vi "Convert DTCs.vi"(11 "value":T2 {"payload" format="%x"; "timestamp" format="%<%.7X\n%x>T"; "type" items=["CAN Data"=0, "CAN Remote"=1, "CAN Bus Error"=2, "CAN 2.0 Data"=8, "CAN FD Data"=16, "CAN FD+BRS Data"=24, "J1939 Data"=192, "Delay"=224, "Log Trigger"=225, "Start Trigger"=226]; "identifier" format="%x"}) -> (3 "Cluster":T1)   [LabVIEW 2015, in "J1939 Addon Shared.lvlib"]
uses:
  J1939 Addon Shared.lvlib
  <vilib>/xnet/xnet.llb/XNET Frame CAN.ctl
  <vilib>/xnet/xnet.llb/XNET Frame Type CAN.ctl
  Types/Convert DTCs Cluster.ctl
  J1939 Utilities/SubVIs/Convert CAN Arb ID to J1939 ID.vi
  J1939 Utilities/J1939 Utilities.lvlib
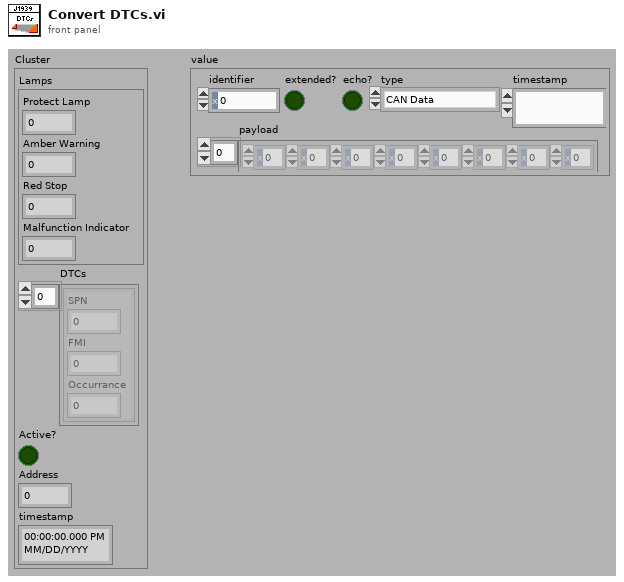
[diagram p1: front panel]
types:
  T1 = typedef "J1939 Addon Shared.lvlib/Convert DTCs Cluster.ctl" = cluster{"Lamps":cluster{"Protect Lamp":u8, "Amber Warning":u8, "Red Stop":u8, "Malfunction Indicator":u8}, "DTCs":cluster{"SPN":u32, "FMI":u8, "Occurrance":u8}[], "Active?":bool, "Address":u8, "timestamp":timestamp}
  T2 = typedef "XNET Frame CAN.ctl" = cluster{"timestamp":timestamp, "payload":u8[], "identifier":u32, "type":T3, "extended?":bool, "echo?":bool}
  T3 = typedef "XNET Frame Type CAN.ctl" = u8
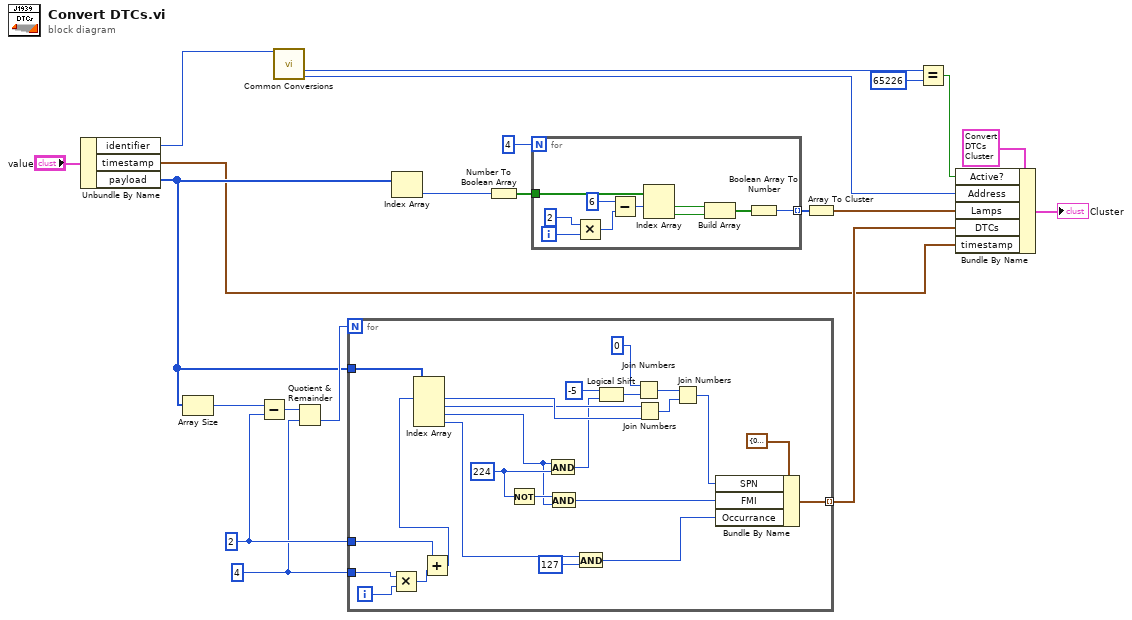
[diagram p0: block diagram]
diagram:
  w10 = 4 ("x")
  w12 = 2 ("x")
  n1 = Unbundle By Name("value") -> ("identifier"=w6:u32, "timestamp"=w1:timestamp, "payload"=w7:u8[])
  n2 = Array Size(array=w7) -> (size(s)=w13:i32)
  n3 = Subtract(x=w13, y=w12) -> (x-y=w11:i32)
  n4 = call-poly "Common Conversions.vi"("Arb ID"=w6) -> ("PGN"=w5:u32, "Source Address"=w2:u8)  [unwired: 11 in, 2 out]
  n5 = Quotient & Remainder(x=w11, y=w10) -> (floor(x/y)=w9:i32)  [unwired: 1 out]
  n6 = for {
    N: w9 -> [_]
    tunnel: w7 -> [w45]
    tunnel: [w30] -> w15 mode=indexing
    tunnel: w12 -> [w26]
    tunnel: w10 -> [w25]
    i -> [w29]
    w39 = u8 224 ("y")
    n7 = Multiply(x=w25, y=w29) -> (x*y=w28:i32)
    n8 = Add(x=w26, y=w28) -> (x+y=w27:i32)
    n9 = Index Array(array=w45, index #1=w27) -> (element #1=w41:u8, element #2=w40:u8, element #3=w37:u8, element #4=w36:u8)  [unwired: 3 in]
    n10 = Not(x=w39) -> (.not. x?=w38:u8)
    n11 = And(x=w37, y=w39) -> (x .and. y?=w23:u8)
    n12 = And(x=w38, y=w37) -> (x .and. y?=w32:u8)
    n13 = And(x=w36, y=u8 127) -> (x .and. y?=w31:u8)
    n14 = Logical Shift(y=i8 -5, x=w23) -> (x << y=w24:u8)
    n15 = Join Numbers(hi=u8 0, lo=w24) -> ((hi.lo)=w43:u16)
    n16 = Join Numbers(hi=w40, lo=w41) -> ((hi.lo)=w42:u16)
    n17 = Join Numbers(hi=w43, lo=w42) -> ((hi.lo)=w33:u32)
    n18 = Bundle By Name(cluster=cluster{"SPN":u32, "FMI":u8, "Occurrance":u8} {"SPN"=0, "FMI"=0, "Occurrance"=0}, "SPN"=w33, "FMI"=w32, "Occurrance"=w31) -> (w30:cluster{"SPN":u32, "FMI":u8, "Occurrance":u8})
  }
  n19 = Index Array(array=w7) -> (element=w19:u8)  [unwired: 1 in]
  n20 = Number To Boolean Array(number=w19) -> (Boolean array=w20:bool[])
  n21 = for {
    N: 4 -> [_]
    tunnel: w20 -> [w55]
    tunnel: [w46] -> w18 mode=indexing
    i -> [w52]
    n22 = Multiply(x=2, y=w52) -> (x*y=w50:i32)
    n23 = Subtract(x=6, y=w50) -> (x-y=w48:i32)
    n24 = Index Array(array=w55, index #1=w48) -> (element #1=w54:bool, element #2=w53:bool)  [unwired: 1 in]
    n25 = Build Array(w54, w53) -> (w47:bool[])
    n26 = Boolean Array To Number(Boolean array=w47) -> (number=w46:u8)
  }
  n27 = Array To Cluster(array=w18) -> (cluster=w16:cluster{"[0]":u8, "[1]":u8, "[2]":u8, "[3]":u8})
  n28 = Equal?(x=w5, y=u32 65226) -> (x = y?=w3:bool)
  n29 = Bundle By Name(cluster=T1 {"Lamps"={"Protect Lamp"=0, "Amber Warning"=0, "Red Stop"=0, "Malfunction Indicator"=0}, "DTCs"=[], "Active?"=FALSE, "Address"=0, "timestamp"=timestamp(0 s since 1904-01-01)} ("Cluster"), "Active?"=w3, "Address"=w2, "Lamps"=w16, "DTCs"=w15, "timestamp"=w1) -> (→"Cluster":T1)
